vi "VISA RS485 WRITE.vi"(7 "error in (no error)":errorcluster, 8 "message":string="p_on", 9 "CIB address":string="e", 10 "VISA resource name":refnum<visa-resource-name>="COM3") -> (0 "error out":errorcluster, 3 "dup VISA resource name":refnum<visa-resource-name>)   [LabVIEW 2013]
doc: "VISA RS485 WRITE ENGINE FOR RTS"
uses:
  <vilib>/Instr/_visa.llb/VISA Flush IO Buffer Mask.ctl
panel:
  out "Sent Message byte length":i32
  out "Transmitted Message byte length":u32
  out "Message Transmitted?":bool
  out "Message Sent":string
  out "Parity set for Messaging mode (SPACE)?":bool
  out "Sent Address byte length":i32
  out "Transmitted Address byte length":u32
  out "Address Transmitted?":bool
  out "Address Sent":string
  out "Parity set for Addressing mode (MARK)?":bool
  # "PORT I/O METHOD INPUT CONTROLS\n              (IN ADDITION TO \n        VISA METHOD CONTROLS)"
  # "VISA METHOD STATUS INDICATORS"
  # "VISA METHOD INPUT CONTROLS"
  # "PORT I/O METHOD STATUS INDICATORS"
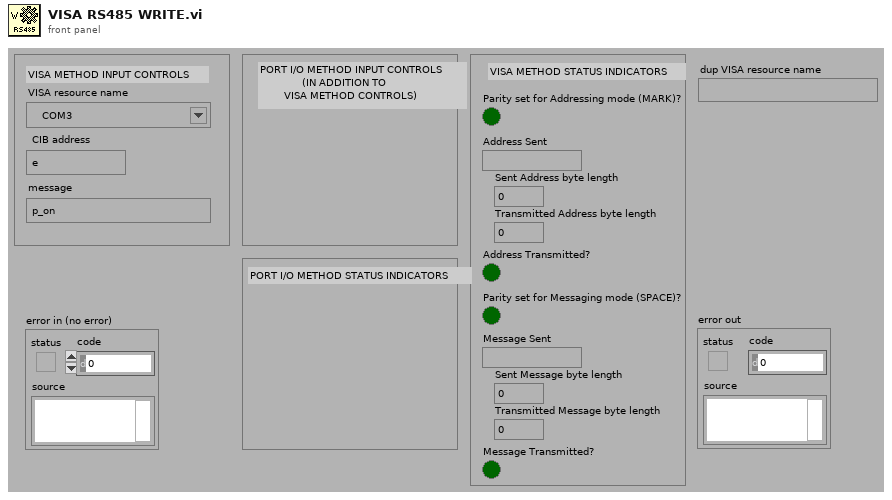
[diagram p1: front panel]
types:
  T1 = typedef "VISA Flush IO Buffer Mask.ctl" = u16
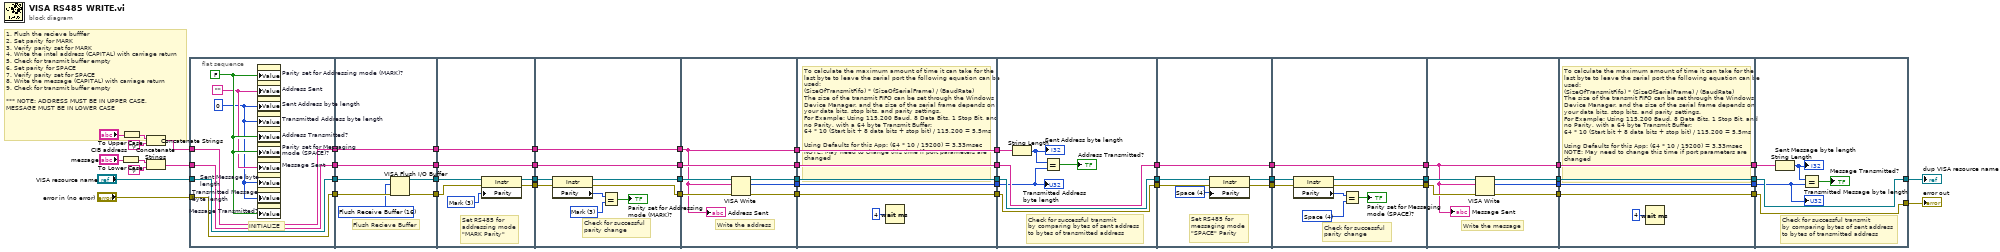
[diagram p0: block diagram]
diagram:
  # "1. Flush the recieve bufffer\n2. Set parity for MARK\n3. Verify parity set for MARK\n4. Write the intel address (CAPITAL) with carriage return\n5. Check for transmit buffer empty\n6. Set parity for SPACE\n7. Verify parity set for SPACE\n8. Write the message (CAPITAL) with carriage return\n9. Check for transmit buffer empty\n\n*** NOTE: ADDRESS MUST BE IN UPPER CASE, \nMESSAGE MUST BE IN LOWER CASE"
  n1 = To Lower Case(string="message") -> (all lower case string=w44:string)
  n2 = To Upper Case(1:"CIB address") -> (0:w45:string)
  n3 = Concatenate Strings(w45, "\r") -> (w52:string)
  n4 = Concatenate Strings(w44, "\r") -> (w50:string)
  n5 = flat-sequence {
    tunnel: "error in (no error)" -> [w57]
    tunnel: "VISA resource name" -> [w56]
    tunnel: w52 -> [w61]
    tunnel: w50 -> [w62]
    tunnel: [w62] -> w43
    tunnel: [w61] -> w42
    tunnel: [w56] -> w41
    tunnel: [w57] -> w40
    tunnel: [w69] -> w39
    tunnel: [w68] -> w38
    tunnel: [w63] -> w37
    tunnel: [w67] -> w36
    tunnel: w43 -> [w69]
    tunnel: w42 -> [w68]
    tunnel: w41 -> [w64]
    tunnel: w40 -> [w66]
    tunnel: w39 -> [w76]
    tunnel: [w76] -> w35
    tunnel: w38 -> [w75]
    tunnel: [w75] -> w34
    tunnel: [w70] -> w33
    tunnel: w37 -> [w71]
    tunnel: w36 -> [w74]
    tunnel: [w72] -> w32
    tunnel: w35 -> [w85]
    tunnel: [w85] -> w31
    tunnel: w34 -> [w84]
    tunnel: [w84] -> w30
    tunnel: [w78] -> w29
    tunnel: w33 -> [w77]
    tunnel: w32 -> [w83]
    tunnel: [w79] -> w28
    tunnel: w31 -> [w92]
    tunnel: [w92] -> w18
    tunnel: w30 -> [w86]
    tunnel: w29 -> [w90]
    tunnel: [w87] -> w16
    tunnel: w28 -> [w89]
    tunnel: [w91] -> w14
    tunnel: [w86] -> w12
    tunnel: [w88] -> w10
    tunnel: w18 -> [w98]
    tunnel: [w98] -> w17
    tunnel: w16 -> [w95]
    tunnel: [w95] -> w15
    tunnel: w14 -> [w94]
    tunnel: [w94] -> w13
    tunnel: w12 -> [w97]
    tunnel: [w97] -> w11
    tunnel: w10 -> [w96]
    tunnel: [w96] -> w9
    tunnel: w17 -> [w105]
    tunnel: [w105] -> w27
    tunnel: w15 -> [w104]
    tunnel: [w104] -> w26
    tunnel: w13 -> [w99]
    tunnel: [w99] -> w25
    tunnel: w11 -> [w103]
    tunnel: w9 -> [w101]
    tunnel: w27 -> [w111]
    tunnel: [w111] -> w24
    tunnel: [w108] -> w23
    tunnel: w26 -> [w106]
    tunnel: w25 -> [w110]
    tunnel: [w107] -> w22
    tunnel: w24 -> [w119]
    tunnel: [w119] -> w21
    tunnel: [w113] -> w20
    tunnel: w23 -> [w114]
    tunnel: w22 -> [w115]
    tunnel: [w112] -> w19
    tunnel: w21 -> [w120]
    tunnel: w20 -> [w125]
    tunnel: [w124] -> w8
    tunnel: w19 -> [w123]
    tunnel: [w120] -> w6
    tunnel: [w122] -> w4
    tunnel: [w121] -> w2
    tunnel: w8 -> [w130]
    tunnel: [w130] -> w7
    tunnel: w6 -> [w129]
    tunnel: [w129] -> w5
    tunnel: w4 -> [w128]
    tunnel: [w128] -> w3
    tunnel: w2 -> [w127]
    tunnel: [w127] -> w1
    tunnel: [w136] -> w49
    tunnel: w7 -> [w136]
    tunnel: w5 -> [w133]
    tunnel: w3 -> [w132]
    tunnel: w1 -> [w131]
    tunnel: [w131] -> w48
    frame #0 {
      w58 = 0 ("Sent Address byte length")
      w59 = ""
      w60 = FALSE ("Parity set for Addressing mode (MARK)?")
      # "INITIALIZE"
      n6 = property on="Parity set for Addressing mode (MARK)?" class="Bool (strict)"("Value"=w60) -> ()  [unwired: 2 in, 2 out]
      n7 = property on="Address Sent" class="Str"("Value"=w59) -> ()  [unwired: 2 in, 2 out]
      n8 = property on="Sent Address byte length" class="DigNum (strict)"("Value"=w58) -> ()  [unwired: 2 in, 2 out]
      n9 = property on="Transmitted Address byte length" class="DigNum (strict)"("Value"=w58) -> ()  [unwired: 2 in, 2 out]
      n10 = property on="Address Transmitted?" class="Bool (strict)"("Value"=w60) -> ()  [unwired: 2 in, 2 out]
      n11 = property on="Parity set for Messaging mode (SPACE)?" class="Bool (strict)"("Value"=w60) -> ()  [unwired: 2 in, 2 out]
      n12 = property on="Message Sent" class="Str"("Value"=w59) -> ()  [unwired: 2 in, 2 out]
      n13 = property on="Sent Message byte length" class="DigNum (strict)"("Value"=w58) -> ()  [unwired: 2 in, 2 out]
      n14 = property on="Transmitted Message byte length" class="DigNum (strict)"("Value"=w58) -> ()  [unwired: 2 in, 2 out]
      n15 = property on="Message Transmitted?" class="Bool (strict)"("Value"=w60) -> ()  [unwired: 2 in, 2 out]
    }
    frame #1 {
      w65 = T1 16 items=["Flush Receive Buffer"=16, "Write Transmit Buffer to Device"=32, "Flush Receive Buffer (No I/O)"=64, "Flush Transmit Buffer"=128] ("Mask")
      # "Flush Recieve Buffer"
      n16 = VISA Flush I/O Buffer(VISA resource name=w64, mask (16)=w65, error in (no error)=w66) -> (VISA resource name out=w63:refnum<visa-resource-name>, error out=w67:errorcluster)
    }
    frame #2 {
      w73 = u16 3 items=["None", "Odd", "Even", "Mark", "Space"] ("Serial Settings:Parity")
      # "Set RS485 for\naddressing mode\n\"MARK Parity\""
      n17 = property class="Instr"(reference=w71, error in=w74, "Parity"=w73) -> (reference out=w70:refnum<visa-resource-name>, error out=w72:errorcluster)
    }
    frame #3 {
      w81 = u16 3 items=["None", "Odd", "Even", "Mark", "Space"] ("Serial Settings:Parity")
      # "Check for successful\nparity change"
      n18 = property class="Instr"(reference=w77, error in=w83) -> (reference out=w78:refnum<visa-resource-name>, error out=w79:errorcluster, "Parity"=w82:u16)
      n19 = Equal?(x=w82, y=w81) -> (x = y?=→"Parity set for Addressing mode (MARK)?":bool)
    }
    frame #4 {
      # "Write the address"
      n20 = VISA Write(VISA resource name=w90, write buffer=w86, error in (no error)=w89) -> (VISA resource name out=w87:refnum<visa-resource-name>, return count=w88:u32, error out=w91:errorcluster)
      "Address Sent" <- w86
    }
    frame #5 {
      # "To calculate the maximum amount of time it can take for the last byte to leave the serial port the following equation can be used:\n(SizeOfTransmitFifo) * (SizeOfSerialFrame) / (BaudRate)\nThe size of the transmit FIFO can be set through the Windows Device Manager, and the size of the serial frame depends on your data bits, stop bits, and parity settings.\nFor Example: Using 115,200 Baud, 8 Data Bits, 1 Stop Bit, and no Parity, with a 64 byte Transmit Buffer:\n64 * 10 (Start bit + 8 data bits + stop bit) / 115,200 = 5.5ms\n\nUsing Defaults for this App: (64 * 10 / 19200) = 3.33msec\nNOTE: May need to change this time if port parameters are changed"
      n21 = Wait (ms)(milliseconds to wait=u32 4) -> ()  [unwired: 1 out]
    }
    frame #6 {
      # "Check for successful transmit\nby comparing bytes of sent address\nto bytes of transmitted address"
      n22 = String Length(string=w103) -> (length=w102:i32)
      "Sent Address byte length" <- w102
      n23 = Equal?(x=w102, y=w101) -> (x = y?=→"Address Transmitted?":bool)
      "Transmitted Address byte length" <- w101
    }
    frame #7 {
      w109 = u16 4 items=["None", "Odd", "Even", "Mark", "Space"] ("Serial Settings:Parity")
      # "Set RS485 for\nmessaging mode\n\"SPACE\" Parity"
      n24 = property class="Instr"(reference=w106, error in=w110, "Parity"=w109) -> (reference out=w108:refnum<visa-resource-name>, error out=w107:errorcluster)
    }
    frame #8 {
      w117 = u16 4 items=["None", "Odd", "Even", "Mark", "Space"] ("Serial Settings:Parity")
      # "Check for successful\nparity change"
      n25 = property class="Instr"(reference=w114, error in=w115) -> (reference out=w113:refnum<visa-resource-name>, error out=w112:errorcluster, "Parity"=w118:u16)
      n26 = Equal?(x=w118, y=w117) -> (x = y?=→"Parity set for Messaging mode (SPACE)?":bool)
    }
    frame #9 {
      # "Write the message"
      n27 = VISA Write(VISA resource name=w125, write buffer=w120, error in (no error)=w123) -> (VISA resource name out=w124:refnum<visa-resource-name>, return count=w122:u32, error out=w121:errorcluster)
      "Message Sent" <- w120
    }
    frame #10 {
      # "To calculate the maximum amount of time it can take for the last byte to leave the serial port the following equation can be used:\n(SizeOfTransmitFifo) * (SizeOfSerialFrame) / (BaudRate)\nThe size of the transmit FIFO can be set through the Windows Device Manager, and the size of the serial frame depends on your data bits, stop bits, and parity settings.\nFor Example: Using 115,200 Baud, 8 Data Bits, 1 Stop Bit, and no Parity, with a 64 byte Transmit Buffer:\n64 * 10 (Start bit + 8 data bits + stop bit) / 115,200 = 5.5ms\n\nUsing Defaults for this App: (64 * 10 / 19200) = 3.33msec\nNOTE: May need to change this time if port parameters are changed"
      n28 = Wait (ms)(milliseconds to wait=u32 4) -> ()  [unwired: 1 out]
    }
    frame #11 {
      # "Check for successful transmit\nby comparing bytes of sent address\nto bytes of transmitted address"
      n29 = String Length(string=w133) -> (length=w135:i32)
      "Sent Message byte length" <- w135
      n30 = Equal?(x=w135, y=w132) -> (x = y?=→"Message Transmitted?":bool)
      "Transmitted Message byte length" <- w132
    }
  }
  "error out" <- w48
  "dup VISA resource name" <- w49
